vi "Process.vi"(0 "reference in":refnum<class "BKP-911x Power Supply.lvclass">, 5 "error in (no error)":errorcluster) -> (14 "reference out":refnum<class "BKP-911x Power Supply.lvclass">, 19 "error out":errorcluster)   [LabVIEW 2018, in "BKP-911x Power Supply.lvclass"]
uses:
  BKP-911x Power Supply.lvclass
  <instrlib>/BK Precision 911X Series/BK Precision 911X Series.lvlib
panel:
  out "Output Enabled":bool
  out "Current Limit (A)":dbl
  out "Voltage Setpoint (V)":dbl
  out "Actual Power Level (W)":dbl format="%.4g"
  out "Actual Current Level (A)":dbl format="%.4g"
  out "Actual Voltage Level (V)":dbl format="%.4g"
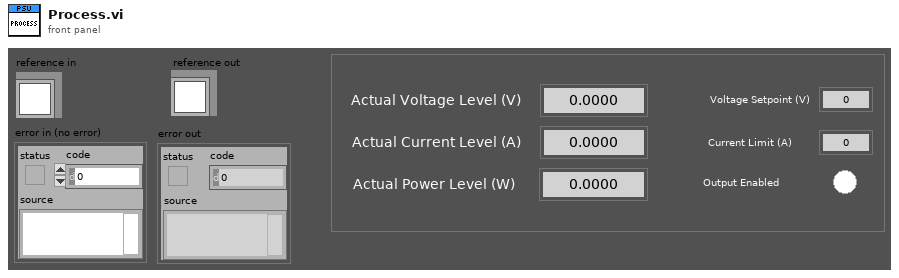
[diagram p1: front panel]
types:
  T1 = cluster{"Event":refnum<event-registration>, "Command":string, "Data":variant}
  T2 = typedef "BKP-911x Power Supply.lvclass/ObjectAttributes.ctl" = cluster{"VISA resource name":refnum<visa-resource-name>, "Simulated?":bool, "Latest Values":dbl[], "Signal List":T3[], "Voltage Setpoint (V)":dbl, "Current Limit (A)":dbl, "Output Enabled?":bool}
  T3 = typedef "IO Signal List.ctl" = enum16{"Timestamp", "PSU_FB_U_VDC", "PSU_FB_I_AMP", "PSU_FB_W_WATT", "PSU_CMD_U_VDC", "PSU_CMD_I_AMP", "PSU_CMD_OUTPUT", "LCR_PRIMARY", "LCR_SECONDARY", "UV_R_mOhm", "UW_R_mOhm", "VW_R_mOhm", "UV_L_µH", "UW_L_µH", "VW_L_µH", "U_U_VDC", "V_U_VDC", "W_U_VDC", "U_I_AMP", "V_I_AMP", "W_I_AMP", "PWM_CMD_DC_%", "PWM_CMD_VDC", "PWM_CMD_Hz", "PWM_FB_DC_%", "PWM_FB_VDC", "PWM_FB_Hz", "DO_RELAY_U_LCR_A", "DO_RELAY_V_LCR_A", "DO_RELAY_V_LCR_B", "DO_RELAY_W_LCR_B", "DIFF_UV_UW_L_µH", "DIFF_UV_VW_L_µH", "DIFF_UW_VW_L_µH", "DIFF_UV_UW_R_mOhm", "DIFF_UV_VW_R_mOhm", "DIFF_UW_VW_R_mOhm", "DIFF_UV_U_VDC", "DIFF_UW_U_VDC", "DIFF_VW_U_VDC"}
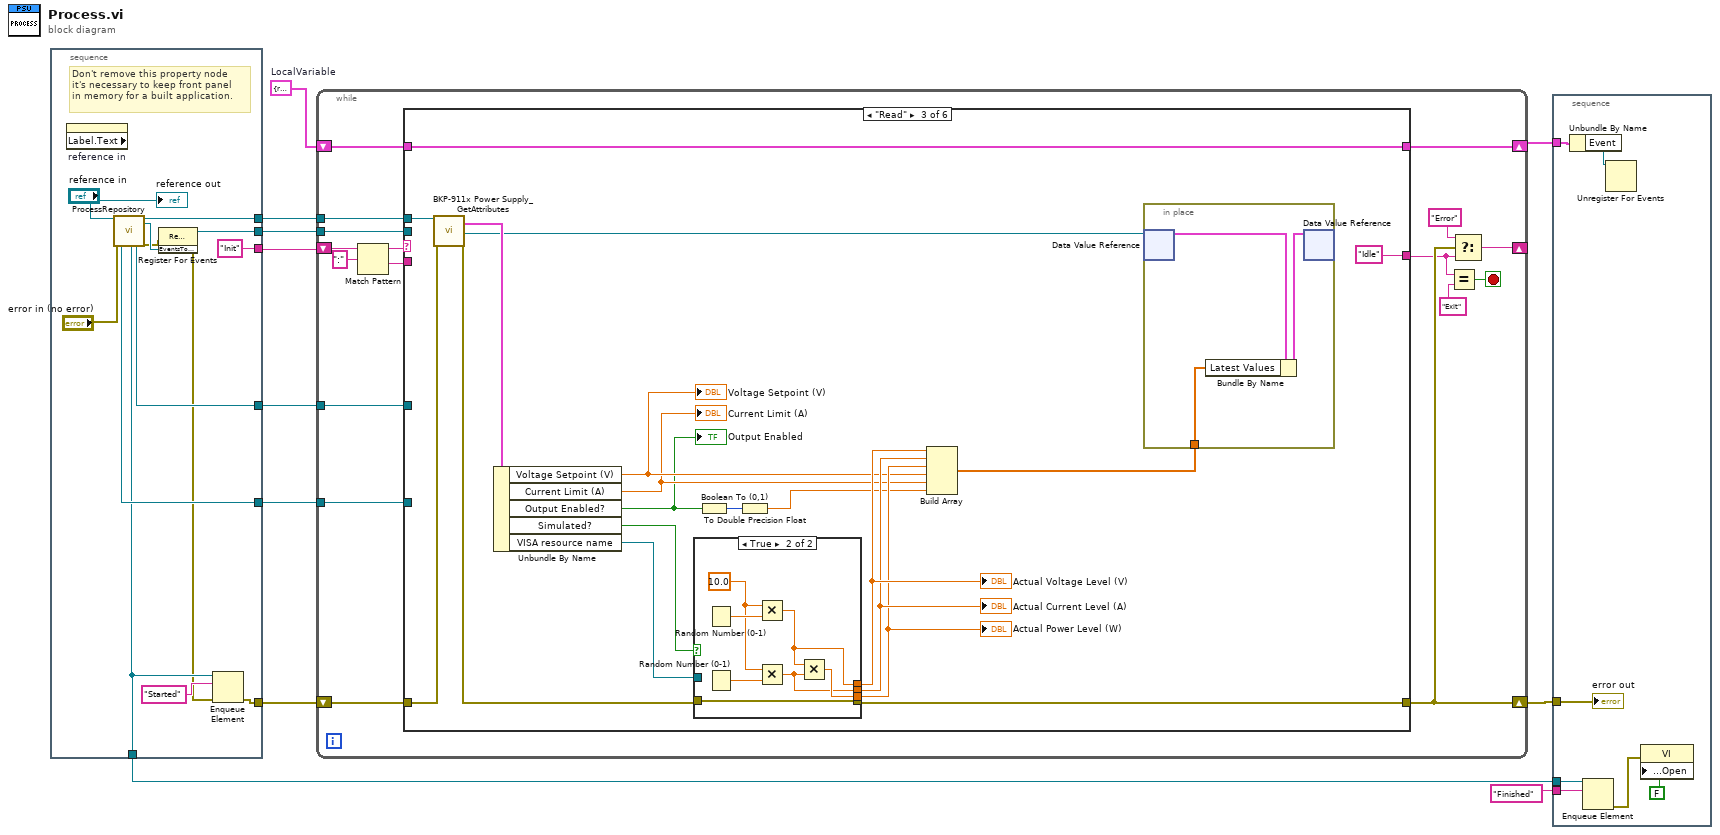
[diagram p0: block diagram]
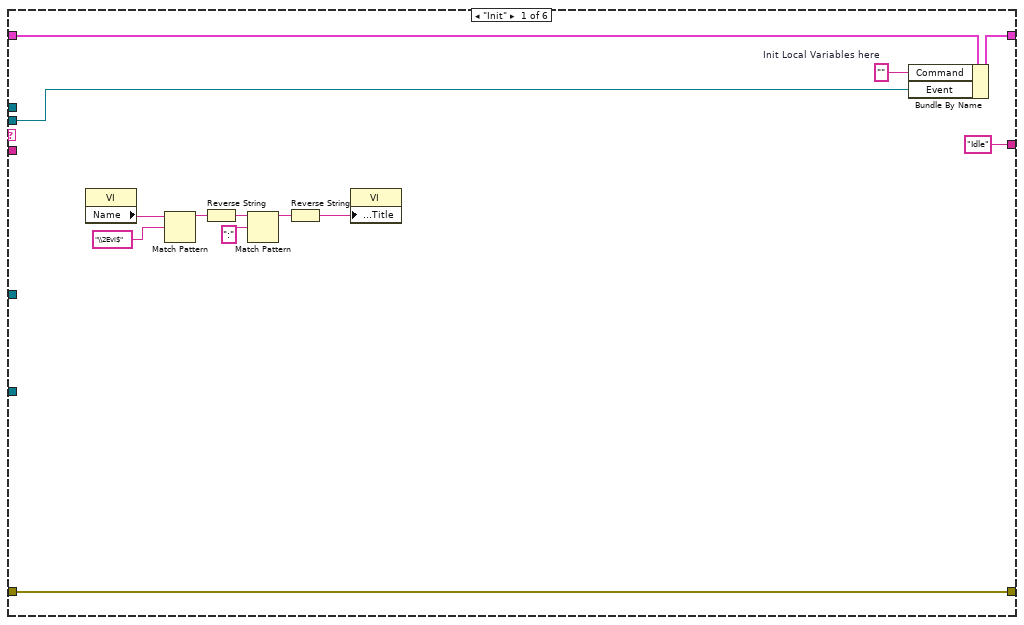
[diagram p2: hidden frame]
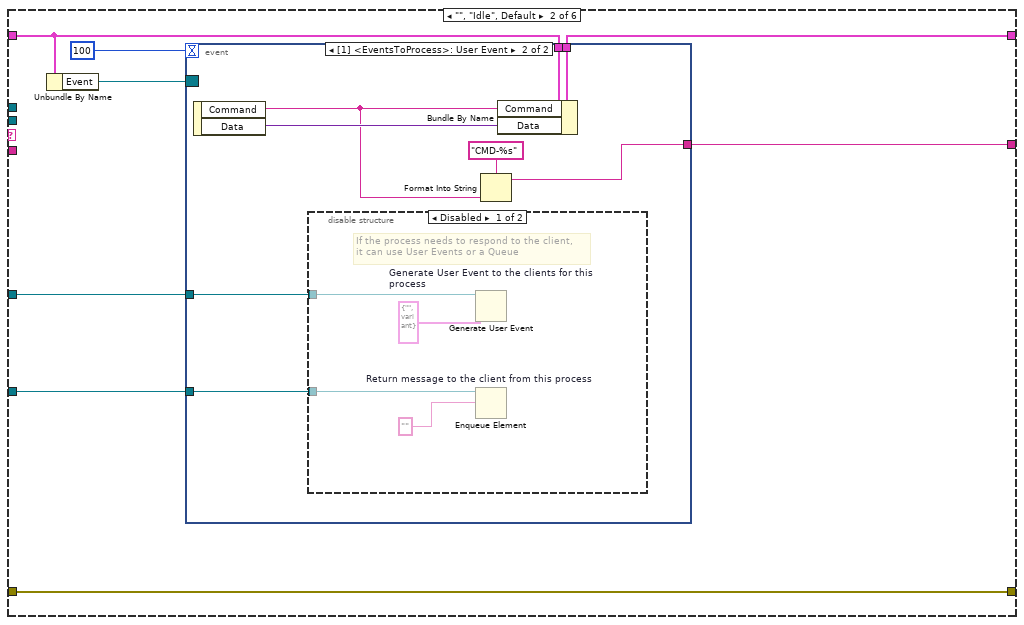
[diagram p3: hidden frame]
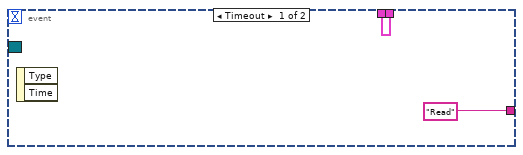
[diagram p4: hidden frame]
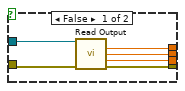
[diagram p6: hidden frame]
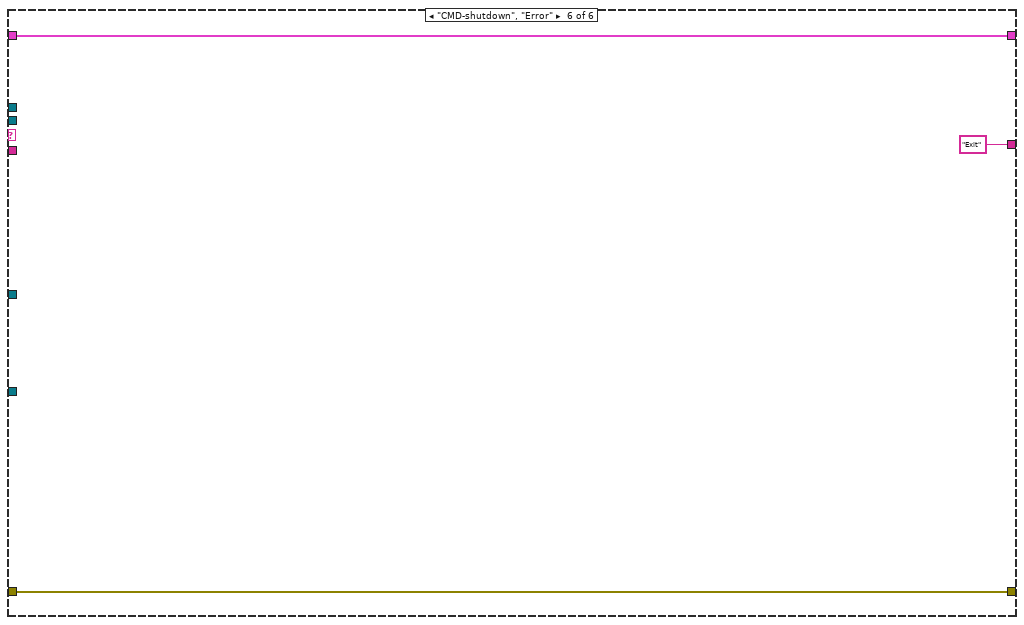
[diagram p9: hidden frame]
diagram:
  w1 = T1 {"Event"=refnum, "Command"="", "Data"=variant}  # LocalVariable
  n1 = stacked-sequence {
    tunnel: [w17] -> w11
    tunnel: [w24] -> w9
    tunnel: [w14] -> w8
    tunnel: [w18] -> w7
    tunnel: ["Init"] -> w6
    tunnel: [w20] -> w4
    tunnel: [w19] -> w3
    frame #0 {
      # "Don't remove this property node\nit's necessary to keep front panel\nin memory for a built application."
      n2 = property on="reference in" class="LVClassControl (strict)" props=["Label", "Text"]() -> ()  [unwired: 2 in, 3 out]
      n3 = call "ProcessRepository.vi"("reference in"="reference in", "error in (no error)"="error in (no error)") -> ("QueueFromProcess"=w19:refnum<queue>, "ProcessSyncQueue"=w18:refnum<queue>, "EventFromProcess"=w20:refnum<user-event>, "reference out"=w24:refnum<class "BKP-911x Power Supply.lvclass">, "EventsToProcess"=w15:refnum<user-event>, "error out"=w13:errorcluster)  [unwired: 10 in, 2 out]
      n4 = register-events(error in=w13, w15) -> (reference out=w14:refnum<event-registration>, error out=w12:errorcluster)  [unwired: 1 in]
      n5 = Enqueue Element(queue=w18, element="Started", error in (no error)=w12) -> (error out=w17:errorcluster)  [unwired: 1 in, 2 out]
      "reference out" <- "reference in"
    }
  }
  n6 = while {
    shift-right: [w34] -> w10
    shift-left: w11 -> [w39]
    tunnel: w9 -> [w40]
    tunnel: w8 -> [w41]
    shift-right: [w32] -> _
    shift-left: w6 -> [w37]
    shift-right: [w28] -> w5
    shift-left: w1 -> [w27]
    tunnel: w4 -> [w26]
    tunnel: w3 -> [w25]
    stop <- w29 stop-if-true
    n7 = Match Pattern(string=w37, regular expression=":") -> (before substring=w36:string, after substring=w35:string)  [unwired: 1 in, 2 out]
    n8 = case shown="\"Read\"" w36 {
      tunnel: w39 -> [w52 w57 w92 w113 w115 w118]
      tunnel: [w52 w57 w89 w113 w115 w118] -> w34
      tunnel: w41 -> [w43 _ _ _ _ _]
      tunnel: w40 -> [_ _ w93 _ _ _]
      tunnel: w35 -> [_ _ _ _ _ _]
      tunnel: ["Idle" ("t") w62 "Idle" ("t") _ _ "Exit" ("y")] -> w31
      tunnel: [w54 w61 w94 w112 w114 w116] -> w28
      tunnel: w27 -> [w42 w60 w94 w112 w114 w116]
      tunnel: w26 -> [_ w56 _ _ _ _]
      tunnel: w25 -> [_ w55 _ _ _ _]
      frame "Init" {
        w53 = ""  # Init Local Variables here
        n9 = property class="VI"() -> ("Name"=w50:string)  [unwired: 2 in, 2 out]
        n10 = Match Pattern(string=w50, regular expression="\\2Evi$") -> (before substring=w48:string)  [unwired: 1 in, 3 out]
        n11 = Reverse String(1:w48) -> (0:w47:string)
        n12 = Match Pattern(string=w47, regular expression=":") -> (before substring=w45:string)  [unwired: 1 in, 3 out]
        n13 = Reverse String(1:w45) -> (0:w44:string)
        n14 = property class="VI"("Front Panel.Title"=w44) -> ()  [unwired: 2 in, 2 out]
        n15 = Bundle By Name(cluster=w42, "Command"=w53, "Event"=w43) -> (w54:T1)
      }
      frame "", "Idle", Default {
        n16 = Unbundle By Name(w60) -> ("Event"=w59:refnum<event-registration>)
        n17 = event shown="[1] <EventsToProcess>: User Event" {
          selector: w59 -> [_ _]
          dyn-events: _ -> [_ _]
          timeout: 100 -> [_ _]
          tunnel: ["Read" ("t") w68] -> w62
          tunnel: w60 -> [w63 w72]
          tunnel: [w63 w71] -> w61
          tunnel: w56 -> [_ w66]
          tunnel: w55 -> [_ w65]
          event Timeout {
            n18 = event-data() -> ()  [unwired: 1 in, 2 out]
          }
          event User Event {
            n19 = event-data() -> ("Command"=w67:string, "Data"=w70:variant)  [unwired: 1 in]
            n20 = disable-structure shown="Disabled" {
              disable-tunnel: w66 -> [w76 _]
              disable-tunnel: w65 -> [w75 _]
              frame Disabled {
                # "If the process needs to respond to the client,\nit can use User Events or a Queue"
                n21 = Generate User Event "Generate User Event to the clients for this process"(user event=w76, event data cluster=cluster{"Command":string, "Data":variant} {"Command"="", "Data"=variant} ("event data")) -> ()  [unwired: 2 in, 2 out]
                n22 = Enqueue Element "Return message to the client from this process"(queue=w75, element="") -> ()  [unwired: 2 in, 3 out]
              }
              frame Enabled {
              }
            }
            n23 = Format Into String(format string="CMD-%s", w67) -> (resulting string=w68:string)  [unwired: 2 in, 1 out]
            n24 = Bundle By Name(cluster=w72, "Command"=w67, "Data"=w70) -> (w71:T1)
          }
        }
      }
      frame "Read" {
        n25 = call "BKP-911x Power Supply_GetAttributes.vi"("reference in"=w93, "error in (no error)"=w92) -> ("Data"=w91:T2, "DataRef"=w85:refnum<data-value>, "error out"=w90:errorcluster)  [unwired: 14 in, 1 out]
        n26 = Unbundle By Name(w91) -> ("Voltage Setpoint (V)"=w83:dbl, "Current Limit (A)"=w82:dbl, "Output Enabled?"=w81:bool, "Simulated?"=w77:bool, "VISA resource name"=w78:refnum<visa-resource-name>)
        "Voltage Setpoint (V)" <- w83
        "Current Limit (A)" <- w82
        "Output Enabled" <- w81
        n27 = case shown="True" w77 {
          tunnel: w90 -> [w101 w108]
          tunnel: [w100 w108] -> w89
          tunnel: w78 -> [w99 _]
          tunnel: [w98 w102] -> w88
          tunnel: [w97 w103] -> w87
          tunnel: [w96 w104] -> w86
          frame False {
            n28 = call <instrlib>:"Read Output.vi"("VISA resource name"=w99, "error in (no error)"=w101) -> ("Actual Voltage Level (V)"=w98:dbl, "Actual Current Level (A)"=w97:dbl, "Actual Power Level (W)"=w96:dbl, "error out"=w100:errorcluster)  [unwired: 8 in, 2 out]
          }
          frame True {
            w105 = 10.0 ("x")
            n29 = Random Number (0-1)() -> (number: 0 to 1=w107:dbl)
            n30 = Random Number (0-1)() -> (number: 0 to 1=w106:dbl)
            n31 = Multiply(x=w105, y=w107) -> (x*y=w102:dbl)
            n32 = Multiply(x=w105, y=w106) -> (x*y=w103:dbl)
            n33 = Multiply(x=w102, y=w103) -> (x*y=w104:dbl)
          }
        }
        "Actual Voltage Level (V)" <- w88
        "Actual Current Level (A)" <- w87
        "Actual Power Level (W)" <- w86
        n34 = Boolean To (0,1)(Boolean=w81) -> (0, 1=w80:i16)
        n35 = To Double Precision Float(number=w80) -> (double precision float=w79:dbl)
        n36 = Build Array(w88, w87, w86, w83, w82, w79) -> (w84:dbl[])
        n37 = in-place {
          in-place-border: w84 -> [w109]
          n38 = in-place-dvr #1(w85) -> (w111:T2)  [unwired: 1 out]
          n39 = Bundle By Name(cluster=w111, "Latest Values"=w109) -> (w110:T2)
          n40 = in-place-dvr #1(w110) -> ()  [unwired: 2 out]
        }
      }
      frame "---- COMMANDS START----" {
      }
      frame "----- COMMANDS END ----" {
      }
      frame "CMD-shutdown", "Error" {
      }
    }
    n41 = Equal?(x=w31, y="Exit") -> (x = y?=w29:bool)
    n42 = Select(t="Error", s=w34, f=w31) -> (s? t:f=w32:string)
  }
  n43 = stacked-sequence {
    tunnel: w10 -> [w125]
    tunnel: w7 -> [w121]
    tunnel: w5 -> [w124]
    tunnel: "Finished" ("element") -> [w119]
    frame #0 {
      n44 = Unbundle By Name(w124) -> ("Event"=w123:refnum<event-registration>)
      n45 = Enqueue Element(queue=w121, element=w119) -> (error out=w120:errorcluster)  [unwired: 2 in, 2 out]
      n46 = Unregister For Events(event registration refnum=w123) -> ()  [unwired: 1 in, 1 out]
      n47 = property class="VI"(error in=w120, "Front Panel.Open"=FALSE ("Front Panel Window:Open")) -> ()  [unwired: 1 in, 2 out]
      "error out" <- w125
    }
  }
